vi "StaticFireVI.vi"() -> ()   [LabVIEW 2016]
uses:
  <vilib>/DAQmx/read.llb/DAQmx Read (Analog 2D DBL NChan NSamp).vi
  <vilib>/DAQmx/miscellaneous.llb/DAQmx Fill In Error Info.vi
  <vilib>/Utility/file.llb/Write To Spreadsheet File (DBL).vi
panel:
  out "Max":dbl
  out "Max":dbl
  out "Max":dbl
  out "Max":dbl
  out ";lj;lkj;lkj 3":dbl
  out ";lj;lkj;lkj 2":dbl
  out ";lj;lkj;lkj":dbl
  out ";lj;lkj;lkj":dbl
  out "Thermocouples 0-3 (Celcius)":cluster{dbl, dbl, dbl, dbl}(knob) caption="Meter" scale=0.0..100.0
  out "Recording 2":bool
  in  "?":bool
  in  "?":bool
  in  "Thermocouple File Path":path=path "C:/Users/Adam/Desktop/OctoberTC.txt"
  in  "Thermocouple Task Name":refnum<k21>="Thermocouples"
  out "Recording":bool
  in  "?":bool
  out "Task Error 2":bool
  out "TC Record Time":dbl format="%<%I:%M:%S%4u %p>T"
  out "PT/LC Record Time":dbl format="%<%I:%M:%S%4u %p>T"
  out "error out 3":errorcluster
  out "Error":bool
  out "Max":dbl
  out "Current":dbl format="%.2f"
  in  "Channel #":dbl=1.0
  out "Pressure Transducer 2":dbl(knob) scale=0.0..1000.0
  in  "Calibration b":dbl
  in  "Calibration a":dbl=200.0
  out "Waveform Chart 3":dbl(graph)
  in  "PT/Load Cell Task Name":refnum<k21>="Load Cell and PTs"
  out "PT Queue Error":bool
  out "Task Error":bool
  out "Time":string
  out "Ch 5":dbl
  in  "Channel 5":i32=5
  out "Ch 4":dbl
  in  "Channel 4":i32=4
  out "Ch 3":dbl format="%<%H:%M:%S>T"
  out "Ch 2":dbl format="%#_6f"
  out "Ch 1":dbl
  out "Ch 0":dbl format="%#_6f"
  in  "Channel 3":i32=3
  in  "Channel 2":i32=2
  in  "Channel 1":i32=1
  in  "Channel 0":i32
  out "Error":bool
  out "Waveform Chart 2":dbl(graph)
  out "Current":dbl format="%#.2f"
  out "Max":dbl
  in  "Channel #":dbl=2.0
  in  "Calibration b":dbl=-0.364
  in  "Calibration a":dbl=1.0
  out "Load Cell":dbl(knob) scale=0.0..500.0
  out "Error":bool
  out "Waveform Chart":dbl(graph)
  out "Current":dbl format="%.2f"
  out "Max":dbl
  in  "Channel #":dbl
  in  "Calibration b":dbl
  in  "Calibration a":dbl=200.0
  out "Pressure Transducer 1":dbl(knob) scale=0.0..1000.0
  in  "PT/Load Cell File Path":path=path "C:/Users/Adam/Desktop/OctoberPTLC.txt"
  in  "?":bool
  # "Calibration Equation\n    PSI = aX + b"
  # "Calibration Equation\n    PSI = aX + b"
  # "Calibration Equation\nPounds = a(X + b)"
  # "TC 1"
  # "TC 2"
  # "TC 3"
  # "TC 4"
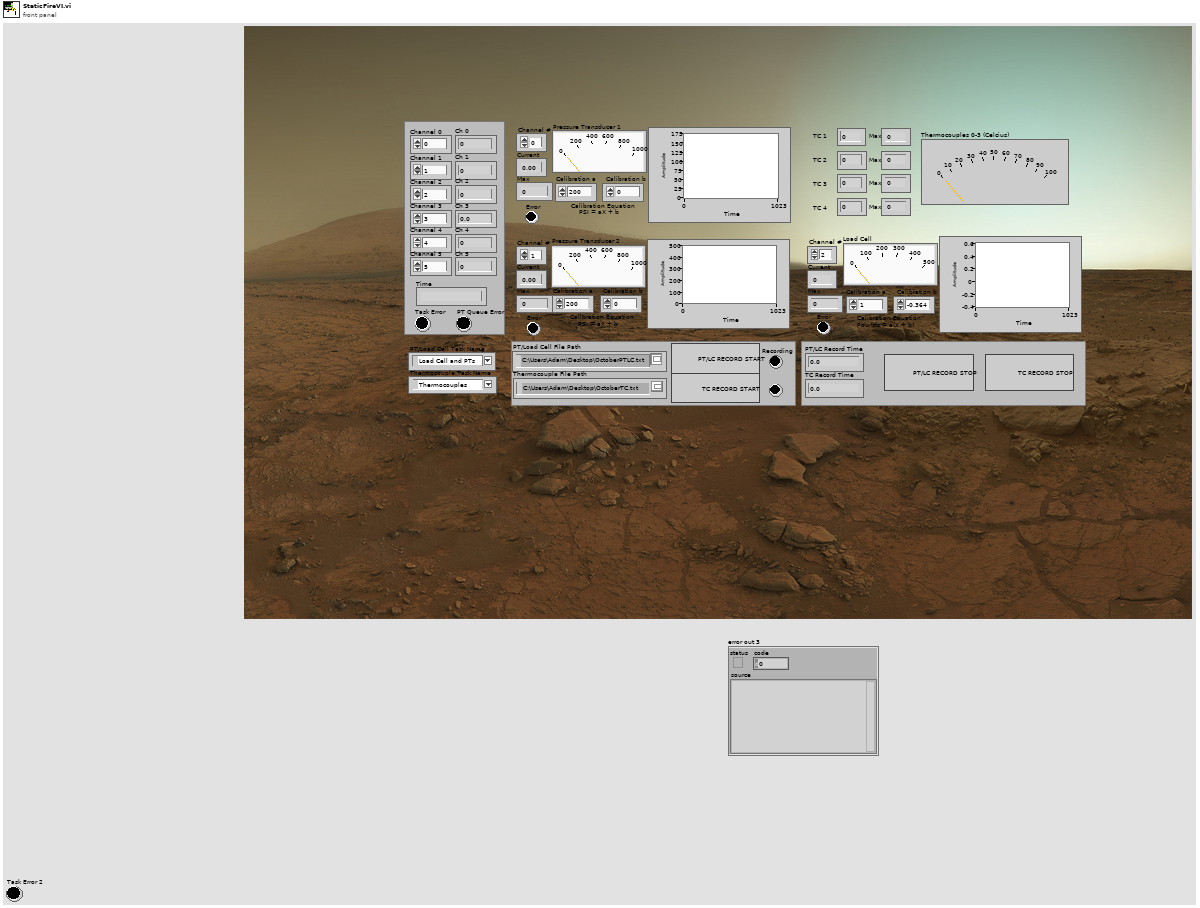
[diagram p1: front panel]
types:
  T1 = cluster{"Waveform":dbl, "Waveform":dbl, "Waveform":dbl, "Waveform":dbl}
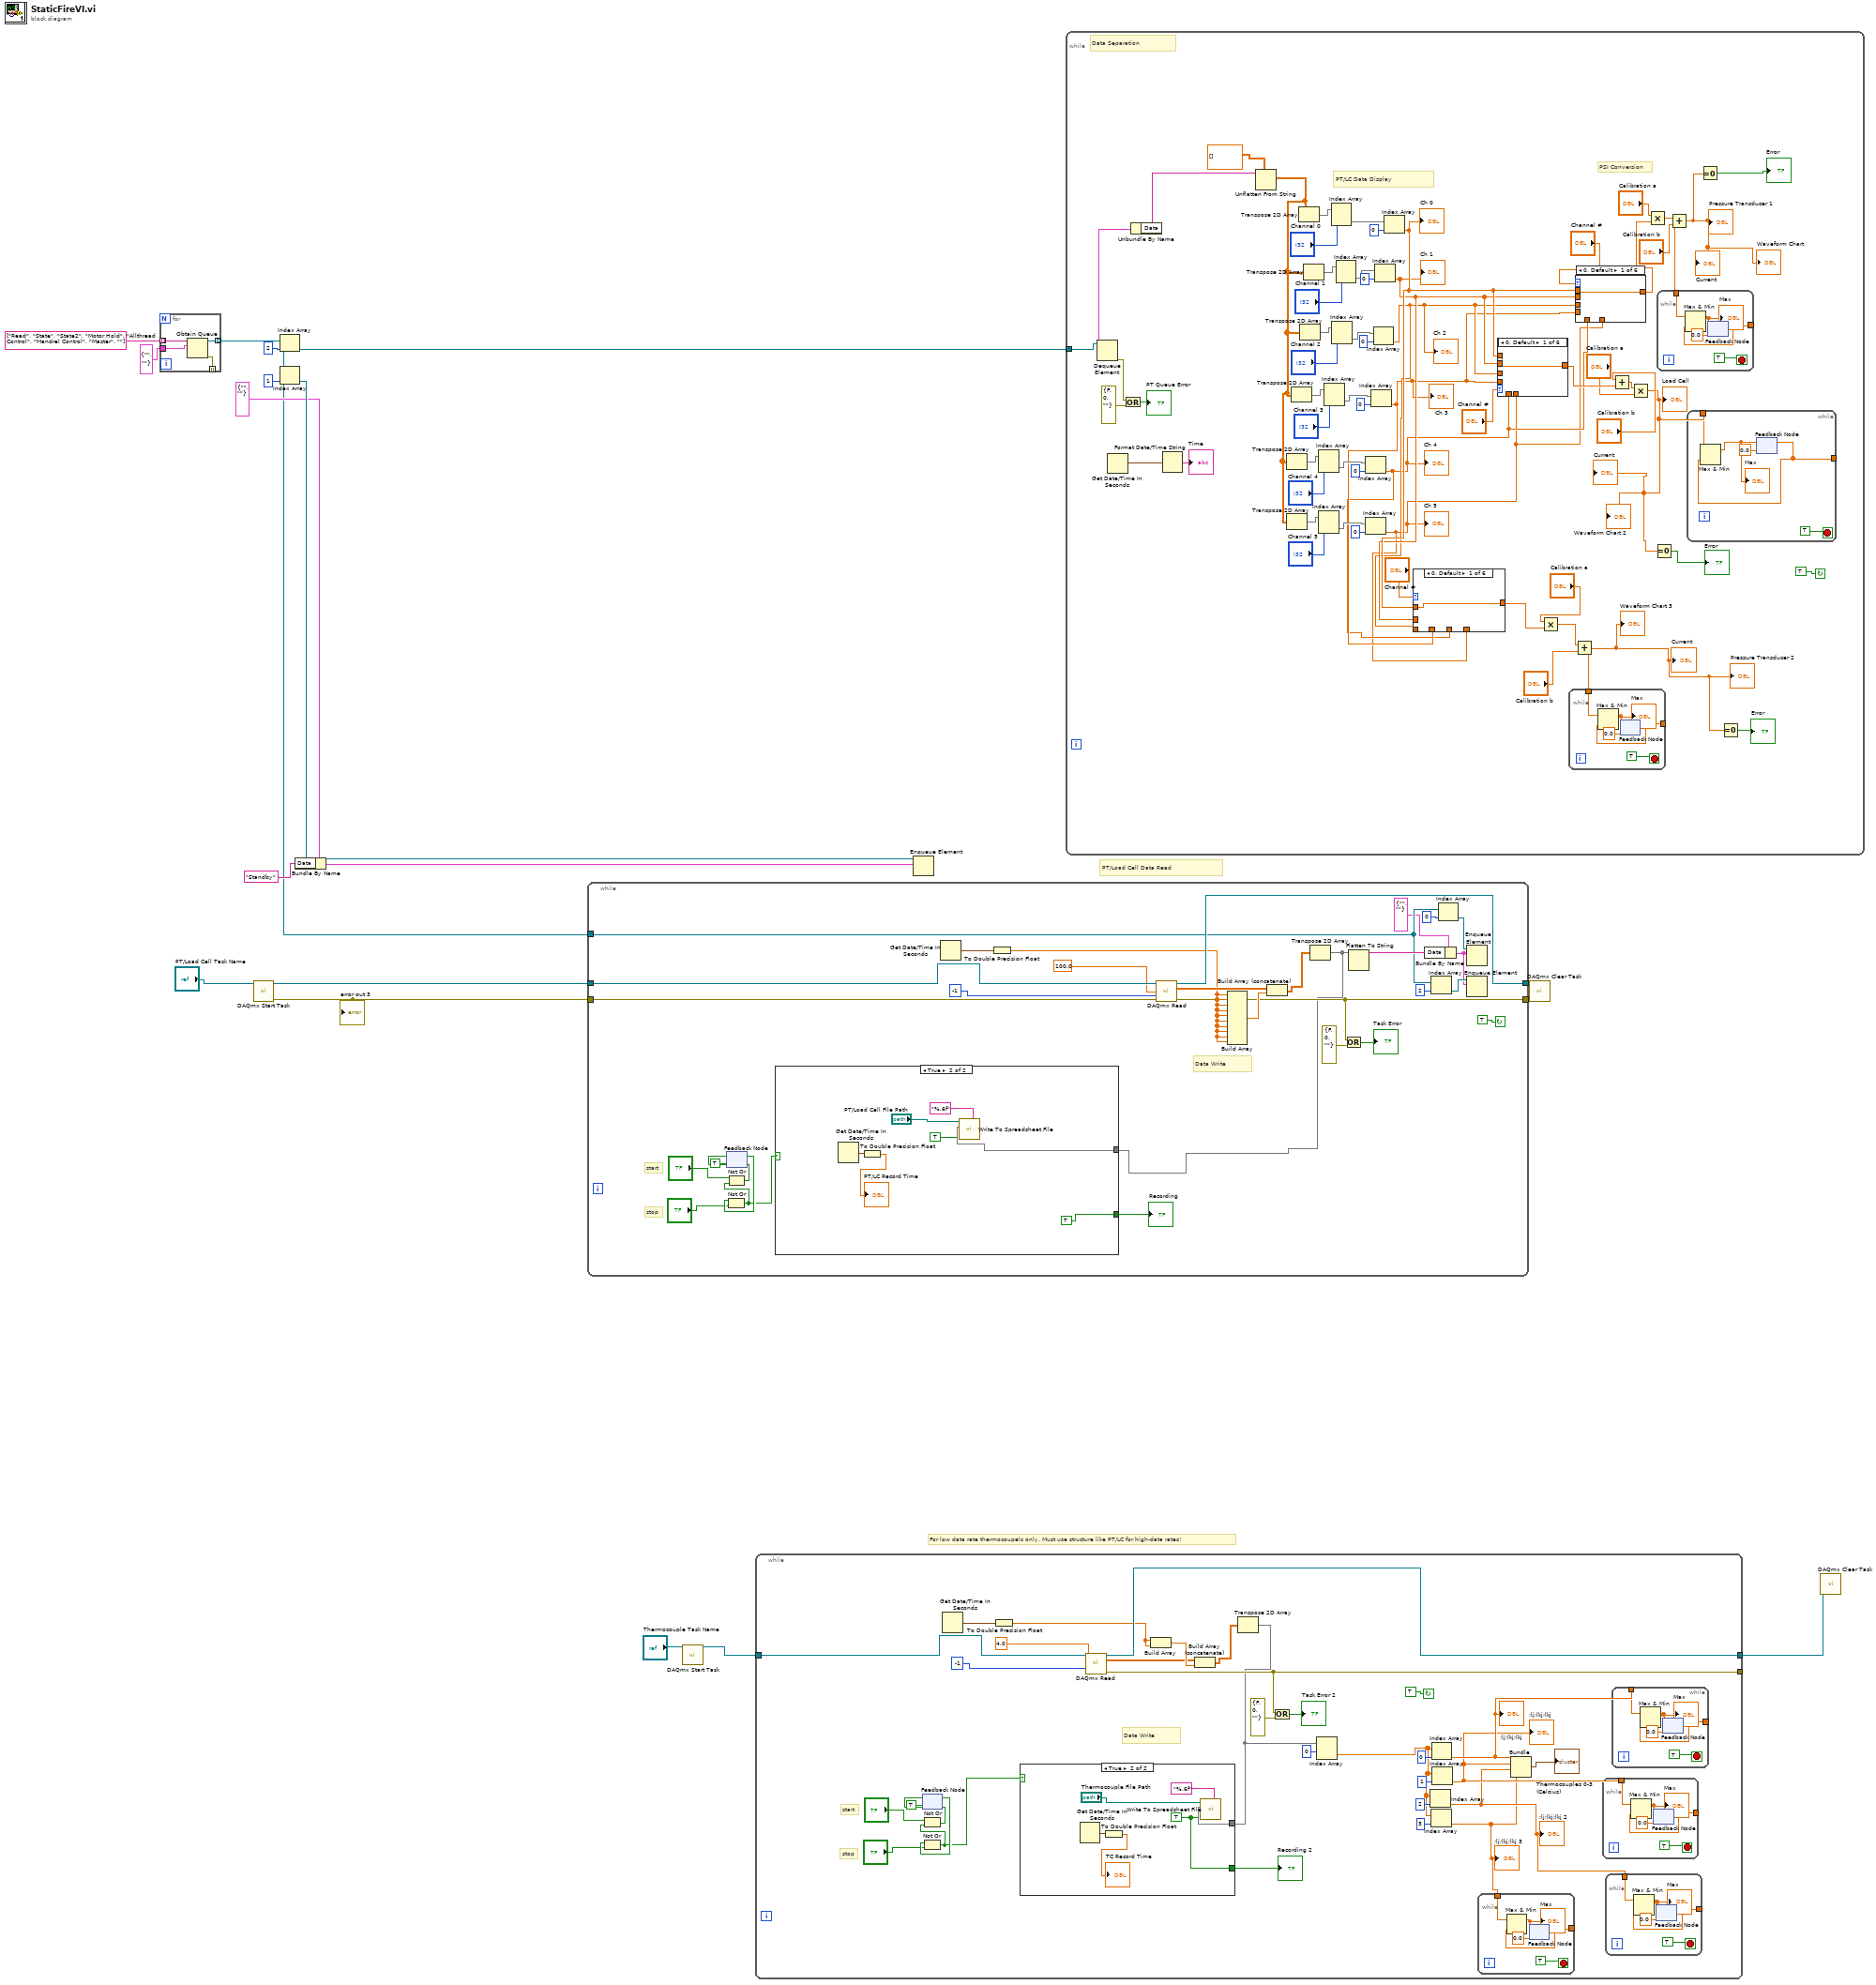
[diagram p0: block diagram]
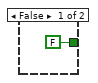
[diagram p2: hidden frame]
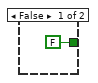
[diagram p18: hidden frame]
diagram:
  # "For low data rate thermocoupels only. Must use structure like PT/LC for high-data rates!"
  # "PT/Load Cell Data Read"
  n1 = for {
    tunnel: string[] ["Read", "State", "State2", "Motor Hold", "Allthread Control", "Mandrel Control", "Master", ""] -> [w22] mode=indexing
    tunnel: [w21] -> w7 mode=indexing
    tunnel: cluster{"Data":string, "State":string} {"Data"="", "State"=""} -> [w20]
    tunnel: [w19] -> _ mode=indexing
    n2 = Obtain Queue(name (unnamed)=w22, element data type=w20) -> (queue out=w21:refnum<queue>, error out=w19:errorcluster)  [unwired: 3 in, 1 out]
  }
  n3 = call <vilib>:"DAQmx Start Task.vi"("task/channels in"="PT/Load Cell Task Name") -> ("task out"=w18:refnum<k21>, "error out"=w17:errorcluster)  [unwired: 13 in]
  "error out 3" <- w17
  n4 = Index Array(array=w7, index=2) -> (element=w8:refnum<queue>)
  n5 = Index Array(array=w7, index=1) -> (element=w13:refnum<queue>)
  n6 = Bundle By Name(cluster=cluster{"Data":string, "State":string} {"Data"="", "State"=""}, "Data"="Standby") -> (w12:cluster{"Data":string, "State":string})
  n7 = while {
    tunnel: w18 -> [w52]
    tunnel: w17 -> [w51]
    tunnel: [w50] -> w6
    tunnel: [w34] -> w5
    tunnel: w7 -> [w46]
    stop <- TRUE continue-if-true
    # "start"
    # "stop"
    # "Data Write"
    n8 = feedback #1(TRUE) -> (w29:bool)
    n9 = Not Or(1:"?", 2:w29) -> (0:w28:bool)
    n10 = Not Or(1:w28, 2:"?") -> (0:w30:bool)
    n11 = feedback-in #1(w30) -> ()
    n12 = Get Date/Time In Seconds() -> (seconds since 1Jan1904=w40:timestamp)
    n13 = To Double Precision Float(number=w40) -> (double precision float=w36:dbl)
    n14 = call-poly <vilib>:"DAQmx Read.vi"("task/channels in"=w52, "number of samples per channel"=100.0, "timeout"=-1 ("number of samples per channel"), "error in"=w51) -> ("task out"=w50:refnum<k21>, "data"=w37:dbl[][], "error out"=w34:errorcluster)  [unwired: 9 in]
    n15 = Build Array(w36, w36, w36, w36, w36, w36, w36, w36, w36, w36) -> (w39:dbl[])
    n16 = Build Array (concatenate)(w37, w39) -> (w32:dbl[][])
    n17 = Transpose 2D Array(2D array=w32) -> (transposed array=w31:dbl[][])
    n18 = case shown="True" w28 {
      tunnel: w31 -> [_ w60]
      tunnel: [FALSE TRUE] -> w27
      frame False {
      }
      frame True {
        n19 = Get Date/Time In Seconds() -> (seconds since 1Jan1904=w56:timestamp)
        n20 = To Double Precision Float(number=w56) -> (double precision float=→"PT/LC Record Time":dbl)
        n21 = call-poly <vilib>:"Write To Spreadsheet File.vi"("format (%.3f)"="%.6f", "append to file? (new file:F)"=TRUE, "2D data"=w60, "file path (dialog if empty)"="PT/Load Cell File Path") -> ()  [unwired: 4 in, 1 out]
      }
    }
    "Recording" <- w27
    n22 = Or(x=w34, y=errorcluster {"status"=FALSE, "code"=0, "source"=""}) -> (x .or. y?=→"Task Error":bool)
    n23 = Flatten To String(anything=w31) -> (data string=w49:string)  [unwired: 3 in, 2 out]
    n24 = Bundle By Name(cluster=cluster{"Data":string, "State":string} {"Data"="", "State"=""}, "Data"=w49) -> (w42:cluster{"Data":string, "State":string})
    n25 = Index Array(array=w46, index=2) -> (element=w43:refnum<queue>)
    n26 = Index Array(array=w46, index=0) -> (element=w44:refnum<queue>)
    n27 = Enqueue Element(queue=w44, element=w42) -> ()  [unwired: 2 in, 3 out]
    n28 = Enqueue Element(queue=w43, element=w42) -> ()  [unwired: 2 in, 3 out]
  }
  n29 = call <vilib>:"DAQmx Start Task.vi"("task/channels in"="Thermocouple Task Name") -> ("task out"=w3:refnum<k21>)  [unwired: 13 in, 1 out]
  n30 = while {
    tunnel: w3 -> [w92]
    tunnel: [w91] -> w2
    tunnel: [w85] -> _
    stop <- TRUE continue-if-true
    # "start"
    # "stop"
    # "Data Write"
    n31 = feedback #2(TRUE) -> (w81:bool)
    n32 = Not Or(1:"?", 2:w81) -> (0:w77:bool)
    n33 = Not Or(1:w77, 2:"?") -> (0:w82:bool)
    n34 = feedback-in #2(w82) -> ()
    n35 = Get Date/Time In Seconds() -> (seconds since 1Jan1904=w88:timestamp)
    n36 = To Double Precision Float(number=w88) -> (double precision float=w87:dbl)
    n37 = call-poly <vilib>:"DAQmx Read.vi"("task/channels in"=w92, "number of samples per channel"=4.0, "timeout"=-1 ("number of samples per channel")) -> ("task out"=w91:refnum<k21>, "data"=w65:dbl[][], "error out"=w85:errorcluster)  [unwired: 10 in]
    n38 = Build Array(w87, w87) -> (w75:dbl[])
    n39 = Build Array (concatenate)(w65, w75) -> (w83:dbl[][])
    n40 = Transpose 2D Array(2D array=w83) -> (transposed array=w64:dbl[][])
    n41 = case shown="True" w77 {
      tunnel: w64 -> [_ w118]
      tunnel: [FALSE ("append to file? (new file:F)") w114] -> w76
      frame False {
      }
      frame True {
        w114 = TRUE ("append to file? (new file:F)")
        n42 = Get Date/Time In Seconds() -> (seconds since 1Jan1904=w117:timestamp)
        n43 = To Double Precision Float(number=w117) -> (double precision float=→"TC Record Time":dbl)
        n44 = call-poly <vilib>:"Write To Spreadsheet File.vi"("format (%.3f)"="%.6f", "append to file? (new file:F)"=w114, "2D data"=w118, "file path (dialog if empty)"="Thermocouple File Path") -> ()  [unwired: 4 in, 1 out]
      }
    }
    "Recording 2" <- w76
    n45 = Or(x=w85, y=errorcluster {"status"=FALSE, "code"=0, "source"=""}) -> (x .or. y?=→"Task Error 2":bool)
    n46 = Index Array(array=w64, index (row)=0) -> (element=w63:dbl[])  [unwired: 1 in]
    n47 = Index Array(array=w63, index=2) -> (element=w67:dbl)
    ";lj;lkj;lkj 2" <- w67
    n48 = Index Array(array=w63, index=3) -> (element=w66:dbl)
    ";lj;lkj;lkj 3" <- w66
    n49 = Index Array(array=w63, index=0) -> (element=w69:dbl)
    ";lj;lkj;lkj" <- w69
    n50 = Index Array(array=w63, index=1) -> (element=w68:dbl)
    ";lj;lkj;lkj" <- w68
    n51 = while {
      tunnel: w66 -> [w97]
      tunnel: [w95] -> _
      stop <- TRUE stop-if-true
      n52 = feedback #3(0.0) -> (w95:dbl)
      n53 = Max & Min(x=w97, y=w95) -> (max(x,y)=w96:dbl)  [unwired: 1 out]
      "Max" <- w96
      n54 = feedback-in #3(w96) -> ()
    }
    n55 = Bundle("Waveform"=w69, "Waveform"=w68, "Waveform"=w67, "Waveform"=w66) -> (→"Thermocouples 0-3 (Celcius)":T1)  [unwired: 1 in]
    n56 = while {
      tunnel: w68 -> [w107]
      tunnel: [w105] -> _
      stop <- TRUE stop-if-true
      n57 = feedback #4(0.0) -> (w105:dbl)
      n58 = Max & Min(x=w107, y=w105) -> (max(x,y)=w106:dbl)  [unwired: 1 out]
      "Max" <- w106
      n59 = feedback-in #4(w106) -> ()
    }
    n60 = while {
      tunnel: w67 -> [w102]
      tunnel: [w100] -> _
      stop <- TRUE stop-if-true
      n61 = feedback #5(0.0) -> (w100:dbl)
      n62 = Max & Min(x=w102, y=w100) -> (max(x,y)=w101:dbl)  [unwired: 1 out]
      "Max" <- w101
      n63 = feedback-in #5(w101) -> ()
    }
    n64 = while {
      tunnel: w69 -> [w112]
      tunnel: [w110] -> _
      stop <- TRUE stop-if-true
      n65 = feedback #6(0.0) -> (w110:dbl)
      n66 = Max & Min(x=w112, y=w110) -> (max(x,y)=w111:dbl)  [unwired: 1 out]
      "Max" <- w111
      n67 = feedback-in #6(w111) -> ()
    }
  }
  n68 = Enqueue Element(queue=w13, element=w12) -> ()  [unwired: 2 in, 3 out]
  n69 = while {
    tunnel: w8 -> [w177]
    stop <- TRUE continue-if-true
    # "PSI Conversion"
    # "PT/LC Data Display"
    # "Data Separation"
    n70 = Dequeue Element(queue=w177) -> (element=w181:cluster{"Data":string, "State":string}, error out=w140:errorcluster)  [unwired: 2 in, 2 out]
    n71 = Get Date/Time In Seconds() -> (seconds since 1Jan1904=w145:timestamp)
    n72 = Or(x=w140, y=errorcluster {"status"=FALSE, "code"=0, "source"=""}) -> (x .or. y?=→"PT Queue Error":bool)
    n73 = Unbundle By Name(w181) -> ("Data"=w180:string)
    n74 = Format Date/Time String(seconds (now)=w145) -> (date/time string=→"Time":string)  [unwired: 2 in]
    n75 = Unflatten From String(type=dbl[][] [], binary string=w180) -> (value=w146:dbl[][])  [unwired: 3 in, 2 out]
    n76 = Transpose 2D Array(2D array=w146) -> (transposed array=w154:dbl[][])
    n77 = Transpose 2D Array(2D array=w146) -> (transposed array=w150:dbl[][])
    n78 = Transpose 2D Array(2D array=w146) -> (transposed array=w170:dbl[][])
    n79 = Transpose 2D Array(2D array=w146) -> (transposed array=w176:dbl[][])
    n80 = Transpose 2D Array(2D array=w146) -> (transposed array=w172:dbl[][])
    n81 = Transpose 2D Array(2D array=w146) -> (transposed array=w174:dbl[][])
    n82 = Index Array(array=w154, index (row)="Channel 4") -> (element=w151:dbl[])  [unwired: 1 in]
    n83 = Index Array(array=w150, index (row)="Channel 5") -> (element=w147:dbl[])  [unwired: 1 in]
    n84 = Index Array(array=w170, index (row)="Channel 3") -> (element=w124:dbl[])  [unwired: 1 in]
    n85 = Index Array(array=w176, index (row)="Channel 0") -> (element=w168:dbl[])  [unwired: 1 in]
    n86 = Index Array(array=w172, index (row)="Channel 2") -> (element=w123:dbl[])  [unwired: 1 in]
    n87 = Index Array(array=w174, index (row)="Channel 1") -> (element=w160:dbl[])  [unwired: 1 in]
    n88 = Index Array(array=w151, index=0) -> (element=w133:dbl)
    "Ch 4" <- w133
    n89 = Index Array(array=w147, index=0) -> (element=w132:dbl)
    "Ch 5" <- w132
    n90 = Index Array(array=w124, index=0) -> (element=w134:dbl)
    "Ch 3" <- w134
    n91 = Index Array(array=w123, index=0) -> (element=w135:dbl)
    "Ch 2" <- w135
    n92 = Index Array(array=w160, index=0) -> (element=w136:dbl)
    "Ch 1" <- w136
    n93 = Index Array(array=w168, index=0) -> (element=w137:dbl)
    "Ch 0" <- w137
    n94 = case shown="0, Default" "Channel #" {
      tunnel: w137 -> [w187 _ _ _ _ _]
      tunnel: w136 -> [_ w188 _ _ _ _]
      tunnel: w135 -> [_ _ w189 _ _ _]
      tunnel: w134 -> [_ _ _ w190 _ _]
      tunnel: w133 -> [_ _ _ _ w191 _]
      tunnel: w132 -> [_ _ _ _ _ w192]
      tunnel: [w187 w188 w189 w190 w191 w192] -> w128
      frame 0, Default {
      }
      frame 1 {
      }
      frame 2 {
      }
      frame 3 {
      }
      frame 4 {
      }
      frame 5 {
      }
    }
    n95 = case shown="0, Default" "Channel #" {
      tunnel: w137 -> [w203 _ _ _ _ _]
      tunnel: w136 -> [_ w204 _ _ _ _]
      tunnel: w135 -> [_ _ w205 _ _ _]
      tunnel: w134 -> [_ _ _ w206 _ _]
      tunnel: [w203 w204 w205 w206 w207 w208] -> w157
      tunnel: w133 -> [_ _ _ _ w207 _]
      tunnel: w132 -> [_ _ _ _ _ w208]
      frame 0, Default {
      }
      frame 1 {
      }
      frame 2 {
      }
      frame 3 {
      }
      frame 4 {
      }
      frame 5 {
      }
    }
    n96 = Multiply(x="Calibration a", y=w128) -> (x*y=w131:dbl)
    n97 = Add(x=w131, y="Calibration b") -> (x+y=w120:dbl)
    "Waveform Chart 3" <- w120
    "Pressure Transducer 2" <- w120
    "Current" <- w120
    n98 = while {
      tunnel: w120 -> [w186]
      tunnel: [w184] -> _
      stop <- TRUE stop-if-true
      n99 = feedback #7(0.0) -> (w184:dbl)
      n100 = Max & Min(x=w186, y=w184) -> (max(x,y)=w185:dbl)  [unwired: 1 out]
      "Max" <- w185
      n101 = feedback-in #7(w185) -> ()
    }
    n102 = case shown="0, Default" "Channel #" {
      tunnel: w137 -> [w209 _ _ _ _ _]
      tunnel: w136 -> [_ w210 _ _ _ _]
      tunnel: w135 -> [_ _ w211 _ _ _]
      tunnel: w134 -> [_ _ _ w212 _ _]
      tunnel: [w209 w210 w211 w212 w213 w214] -> w155
      tunnel: w133 -> [_ _ _ _ w213 _]
      tunnel: w132 -> [_ _ _ _ _ w214]
      frame 0, Default {
      }
      frame 1 {
      }
      frame 2 {
      }
      frame 3 {
      }
      frame 4 {
      }
      frame 5 {
      }
    }
    n103 = Add(x="Calibration b", y=w157) -> (x+y=w158:dbl)
    n104 = Multiply(x=w158, y="Calibration a") -> (x*y=w121:dbl)
    "Load Cell" <- w121
    "Current" <- w121
    "Waveform Chart 2" <- w121
    n105 = Multiply(x="Calibration a", y=w155) -> (x*y=w165:dbl)
    n106 = Equal To 0?(x=w121) -> (x = 0?=→"Error":bool)
    n107 = Add(x=w165, y="Calibration b") -> (x+y=w122:dbl)
    "Pressure Transducer 1" <- w122
    "Current" <- w122
    "Waveform Chart" <- w122
    n108 = while {
      tunnel: w122 -> [w202]
      tunnel: [w200] -> _
      stop <- TRUE stop-if-true
      n109 = feedback #8(0.0) -> (w200:dbl)
      n110 = Max & Min(x=w202, y=w200) -> (max(x,y)=w201:dbl)  [unwired: 1 out]
      "Max" <- w201
      n111 = feedback-in #8(w201) -> ()
    }
    n112 = while {
      tunnel: w121 -> [w196]
      tunnel: [w195] -> _
      stop <- TRUE stop-if-true
      n113 = feedback #9(0.0) -> (w195:dbl)
      n114 = Max & Min(x=w196, y=w195) -> (max(x,y)=w194:dbl)  [unwired: 1 out]
      "Max" <- w194
      n115 = feedback-in #9(w194) -> ()
    }
    n116 = Equal To 0?(x=w122) -> (x = 0?=→"Error":bool)
    n117 = Equal To 0?(x=w120) -> (x = 0?=→"Error":bool)
  }
  n118 = call <vilib>:"DAQmx Clear Task.vi"("task in"=w6, "error in"=w5) -> ()  [unwired: 13 in, 1 out]
  n119 = call <vilib>:"DAQmx Clear Task.vi"("task in"=w2) -> ()  [unwired: 14 in, 1 out]
